vi "Create New Object.vi"(4 "Error In":errorcluster) -> (0 "Error Out":errorcluster, 3 "Config Data":refnum<class "Config Data.lvclass">)   [LabVIEW 2020, in "Config Data.lvlib" / "Config Data.lvclass"]
uses:
  Config Data.lvclass
  Config Data.lvclass/Config Data.ctl
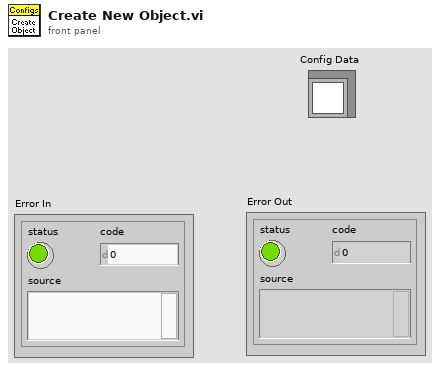
[diagram p1: front panel]
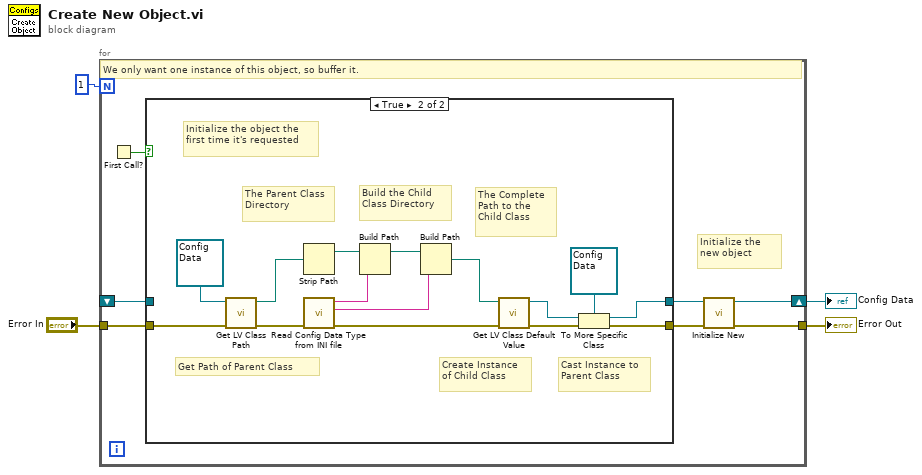
[diagram p0: block diagram]
diagram:
  n1 = for {
    N: 1 -> [_]
    tunnel: "Error In" -> [w11]
    tunnel: [w6] -> w2
    shift-right: [w5] -> w3
    shift-left: _ -> [w10]
    # "Initialize the new object"
    # "We only want one instance of this object, so buffer it."
    n2 = First Call?() -> (First Call?: T/F=w9:bool)
    n3 = case shown="True" w9 {
      tunnel: w11 -> [w12 w28]
      tunnel: [w13 w15] -> w8
      tunnel: [w12 w14] -> w7
      tunnel: w10 -> [w13 _]
      frame False {
      }
      frame True {
        # "Build the Child Class Directory"
        # "The Parent Class Directory"
        # "Initialize the object the first time it's requested"
        # "Cast Instance to Parent Class"
        # "Create Instance of Child Class"
        # "The Complete Path to the Child Class"
        # "Get Path of Parent Class"
        n4 = call <vilib>:"Get LV Class Path.vi"("error in (no error)"=w28, "object"=refnum<class "Config Data.lvclass"> refnum ("Launch Items")) -> ("error out"=w25:errorcluster, "class path"=w21:path)  [unwired: 8 in]
        n5 = Strip Path(path=w21) -> (stripped path=w20:path)  [unwired: 1 out]
        n6 = call "Read Config Data Type from INI file.vi"("Error In"=w25) -> ("Error Out"=w24:errorcluster, "subclass name"=w17:string, "subclass relative path"=w19:string)  [unwired: 4 in]
        n7 = Build Path(base path=w20, name or relative path=w19) -> (appended path=w18:path)
        n8 = Build Path(base path=w18, name or relative path=w17) -> (appended path=w16:path)
        n9 = call <vilib>:"Get LV Class Default Value.vi"("error in (no error)"=w24, "class path"=w16) -> ("error out"=w27:errorcluster, "object"=w26:refnum<class>)  [unwired: 8 in]
        n10 = To More Specific Class(target class=refnum<class "Config Data.lvclass"> refnum ("Launch Items"), reference=w26, error in=w27) -> (specific class reference=w15:refnum<class "Config Data.lvclass">, error out=w14:errorcluster)
      }
    }
    n11 = call-dynamic "Initialize New.vi"("Error In"=w7, "Config Data in"=w8) -> ("Error Out"=w6:errorcluster, "Config Data out"=w5:refnum<class "Config Data.lvclass">)  [unwired: 4 in]
  }
  "Error Out" <- w2
  "Config Data" <- w3
